vi "Set JSON Array.vi"(8 "error in (no error)":errorcluster, 10 "Array":refnum<class "JSON Value.lvclass">[](array[class]), 11 "JSON Array in":refnum<class "JSON Array.lvclass">) -> (0 "error out":errorcluster, 3 "JSON Array out":refnum<class "JSON Array.lvclass">)   [LabVIEW 2020, in "Library Commun.lvlib" / "JSON Array.lvclass"]
uses:
  JSON Array.lvclass
  JSON Value/JSON Value.lvclass
  JSON Array.lvclass/JSON Array.ctl
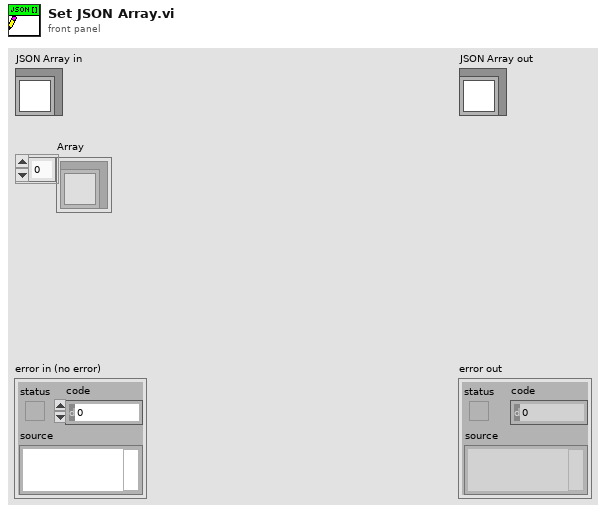
[diagram p1: front panel]
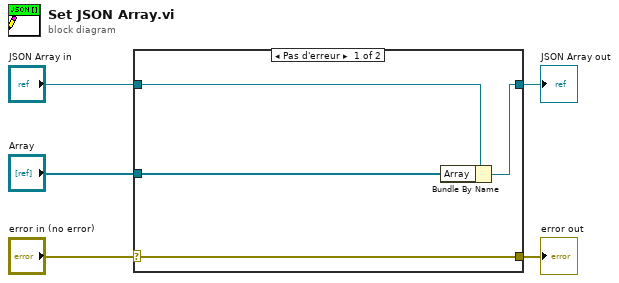
[diagram p0: block diagram]
diagram:
  n1 = case shown="Pas d'erreur" "error in (no error)" {
    selector: "error in (no error)" -> [w9 w10]
    tunnel: [w9 w10] -> w4
    tunnel: [w7 w11] -> w2
    tunnel: "JSON Array in" -> [w8 w11]
    tunnel: "Array" -> [w6 _]
    frame No Error {
      n2 = Bundle By Name(cluster=w8, "Array"=w6) -> (w7:refnum<class "JSON Array.lvclass">)
    }
    frame Error {
    }
  }
  "error out" <- w4
  "JSON Array out" <- w2
